vi "SetWindowAspectRatio.vi"(8 "No Error":errorcluster, 9 "Max Aspect":sgl, 10 "Min Aspect":sgl, 11 "Window [SDL_Window *]":i64 format="%.0x") -> (0 "Error Out":errorcluster)   [LabVIEW 2024, in "SDL3.lvlib" / "Video.lvlib"]
doc: "<B>Summary</B>\nRequest that the aspect ratio of a window's client area be set.\n\n<B>Remarks</B>\nThe aspect ratio is the ratio of width divided by height, e.g. 2560x1600 would be 1.6. Larger aspect ratios are wider and smaller aspect ratios are narrower.\n\nIf, at the time of this request, the window in a fixed-size state, such as maximized or fullscreen, the request will be deferred until the window exits this state and becomes resizable again.\n\nOn some windowing systems, this request is asynchronous and the new window aspect ratio may not have have been applied immediately upon the return of this function. If an immediate change is required, call <B>SDL_SyncWindow()</B> to block until the changes have taken effect.\n\nWhen the window size changes, an <B>SDL_EVENT_WINDOW_RESIZED</B> event will be emitted with the new window dimensions. Note that the new dimensions may not match the exact aspect ratio requested, as some windowing systems can restrict the window size in certain scenarios (e.g. constraining the size of the content area to remain within the usable desktop bounds). Additionally, as this is just a request, it can be denied by the windowing system."
uses:
  Video.lvlib
  Error/Error.lvlib
  Lib/SDL3-32.dll
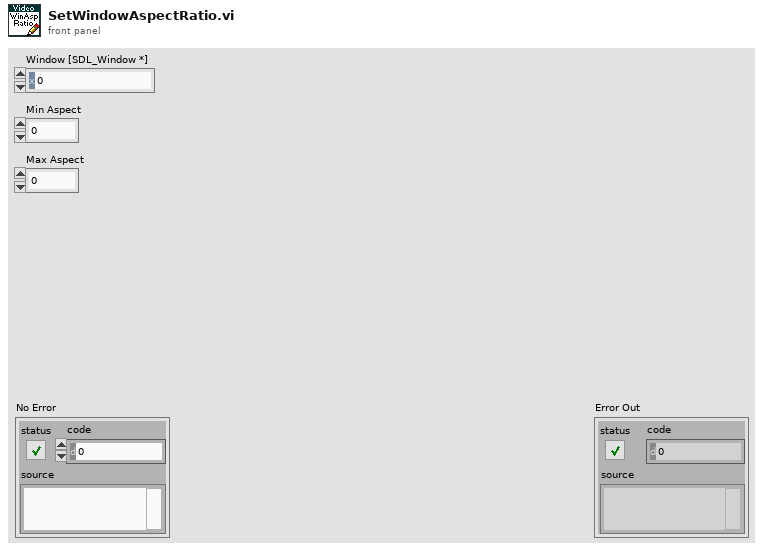
[diagram p1: front panel]
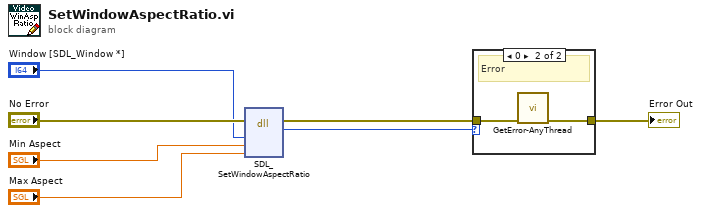
[diagram p0: block diagram]
diagram:
  n1 = dll-call lib="C:/Users/Thomas/Documents/Projects/LV-SDL3/Lib/SDL3-*.*" fn="SDL_SetWindowAspectRatio"(error in="No Error", "window"="Window [SDL_Window *]", "min_aspect"="Min Aspect", "max_aspect"="Max Aspect") -> (error out=w4:errorcluster, "return type"=w3:i32)  [unwired: 5 in, 1 out]
  n2 = case shown="0" w3 {
    tunnel: w4 -> [w8 w10]
    tunnel: [w8 w9] -> w6
    frame Default {
      # "Ok"
    }
    frame 0 {
      # "Error"
      n3 = call "GetError-AnyThread.vi"("No Error"=w10) -> ("Error Out"=w9:errorcluster)  [unwired: 10 in]
    }
  }
  "Error Out" <- w6
